vi "Clear Listeners.vi"(8 "Error In":errorcluster, 11 "Listeners In":refnum<queue>[](array[refnum])) -> (0 "Error Out":errorcluster, 3 "Listeners Out":refnum<queue>[](array[refnum]))   [LabVIEW 2025, in "LOGlib_LV2025.lvlib"]
uses:
  LOGlib_LV2025.lvlib
  Type Definitions/Statement.ctl
  Type Definitions/Tag.ctl
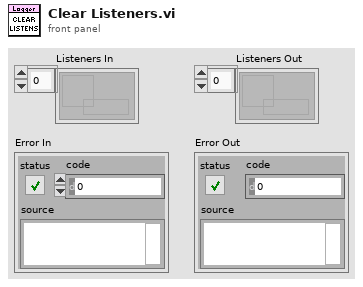
[diagram p1: front panel]
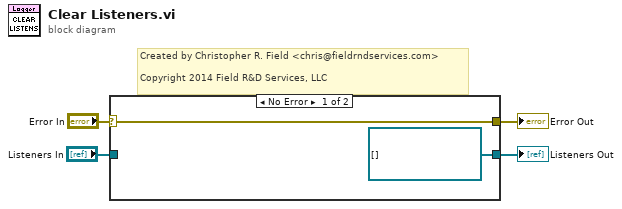
[diagram p0: block diagram]
diagram:
  # "Created by Christopher R. Field <chris@fieldrndservices.com>\n\nCopyright 2014 Field R&D Services, LLC"
  n1 = case shown="No Error" "Error In" {
    selector: "Error In" -> [w5 w7]
    tunnel: [refnum<queue>[] [] w8] -> w4
    tunnel: "Listeners In" -> [_ w8]
    tunnel: [w5 w7] -> w1
    frame No Error {
    }
    frame Error {
    }
  }
  "Listeners Out" <- w4
  "Error Out" <- w1
